vi "Update New Plugin Control.vi"(8 "error in (no error)":errorcluster, 10 "Plugin Types Tree":refnum<vi>, 11 "New Plugin Control":refnum<vi>) -> (0 "error out":errorcluster)   [LabVIEW 2021, in "CIF_UI.lvclass"]
uses:
  CIF_UI.lvclass
  Typedef/New Plugin.ctl
  CIF_UI.lvclass/CIF_UI.ctl
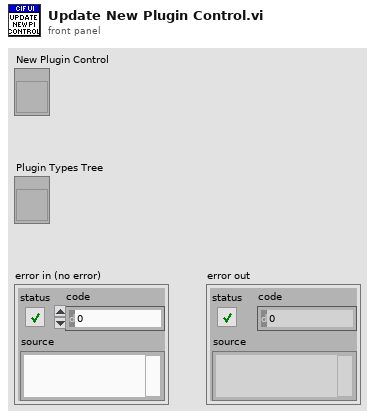
[diagram p1: front panel]
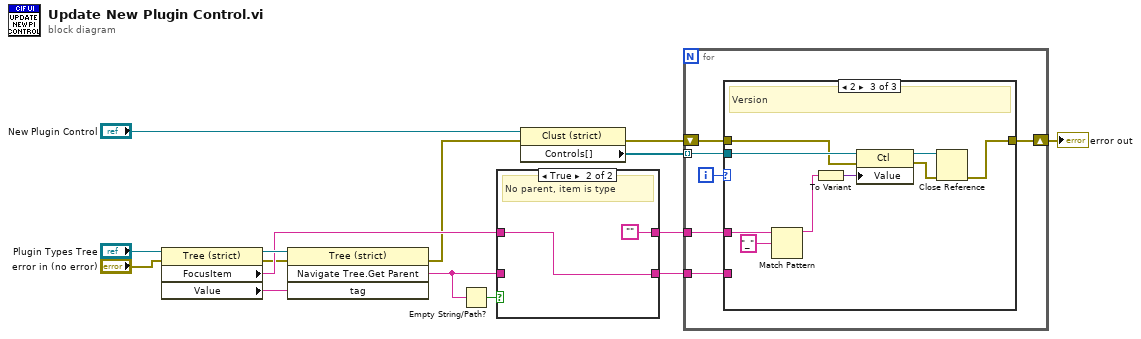
[diagram p0: block diagram]
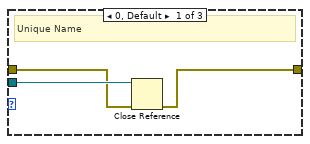
[diagram p3: hidden frame]
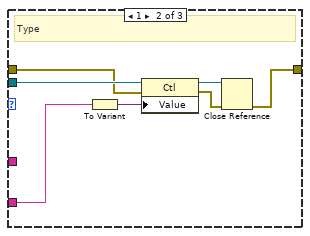
[diagram p4: hidden frame]
diagram:
  n1 = property class="Tree (strict)"(reference="Plugin Types Tree", error in="error in (no error)") -> (error out=w7:errorcluster, "FocusItem"=w8:string, "Value"=w13:string)  [unwired: 1 out]
  n2 = invoke class="Tree (strict)" method="Navigate Tree.Get Parent"(reference="Plugin Types Tree", error in=w7, "tag"=w13) -> (error out=w6:errorcluster, "Navigate Tree:Get Parent"=w9:string)  [unwired: 1 in, 2 out]
  n3 = Empty String/Path?(string/path=w9) -> (empty?=w10:bool)
  n4 = case shown="True" w10 {
    tunnel: w9 -> [w15 _]
    tunnel: w8 -> [w16 w18]
    tunnel: [w16 ""] -> w4
    tunnel: [w15 w18] -> w5
    frame False {
      # "Parent is type, item is version"
    }
    frame True {
      # "No parent, item is type"
    }
  }
  n5 = property class="Clust (strict)"(reference="New Plugin Control", error in=w6) -> (error out=w3:errorcluster, "Controls[]"=w14:refnum<vi>[])  [unwired: 1 out]
  n6 = for {
    tunnel: w14 -> [w23] mode=indexing
    tunnel: w5 -> [w22]
    tunnel: w4 -> [w21]
    shift-right: [w19] -> w1
    shift-left: w3 -> [w20]
    i -> [w24]
    n7 = case shown="2" w24 {
      tunnel: w23 -> [w27 w34 w43]
      tunnel: w22 -> [_ w32 _]
      tunnel: w21 -> [_ _ w37]
      tunnel: w20 -> [w26 w31 w41]
      tunnel: [w25 w28 w38] -> w19
      frame 0, Default {
        # "Unique Name"
        n8 = Close Reference(reference=w27, error in (no error)=w26) -> (error out=w25:errorcluster)
      }
      frame 1 {
        # "Type"
        n9 = To Variant(anything=w32) -> (Variant=w33:variant)
        n10 = property class="Ctl"(reference=w34, error in=w31, "Value"=w33) -> (reference out=w30:refnum<vi>, error out=w29:errorcluster)
        n11 = Close Reference(reference=w30, error in (no error)=w29) -> (error out=w28:errorcluster)
      }
      frame 2 {
        # "Version"
        n12 = Match Pattern(string=w37, regular expression="_") -> (before substring=w35:string)  [unwired: 1 in, 3 out]
        n13 = To Variant(anything=w35) -> (Variant=w42:variant)
        n14 = property class="Ctl"(reference=w43, error in=w41, "Value"=w42) -> (reference out=w40:refnum<vi>, error out=w39:errorcluster)
        n15 = Close Reference(reference=w40, error in (no error)=w39) -> (error out=w38:errorcluster)
      }
    }
  }
  "error out" <- w1
